vi "svl_Maximum Sound Level (1 Ch).vi"(6 "restart averaging (F)":bool, 8 "error in (no error)":errorcluster, 11 "energy level [dB]":waveform(dbl)={"t0"=timestamp(0 s since 1904-01-01), "dt"=0.0, "Y"=[]}) -> (0 "error out":errorcluster, 3 "maximum sound level [dB EU]":dbl format="%.2f")   [LabVIEW 2017]
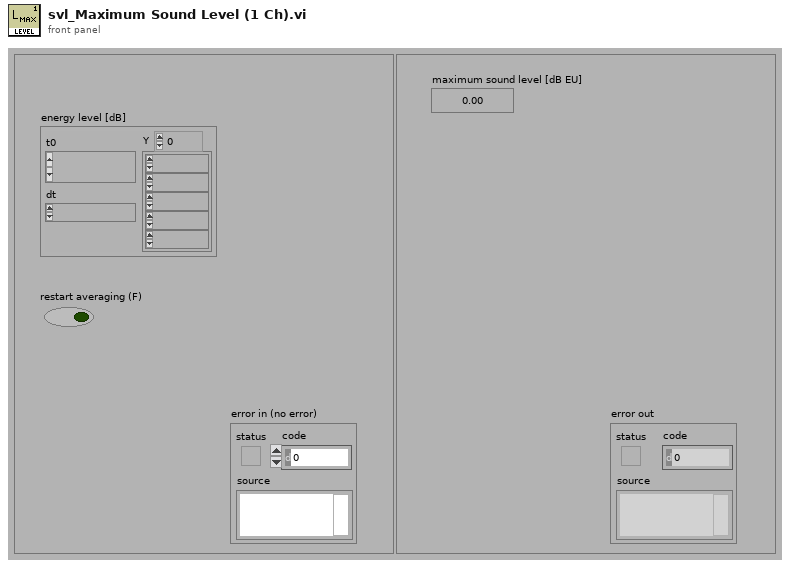
[diagram p1: front panel]
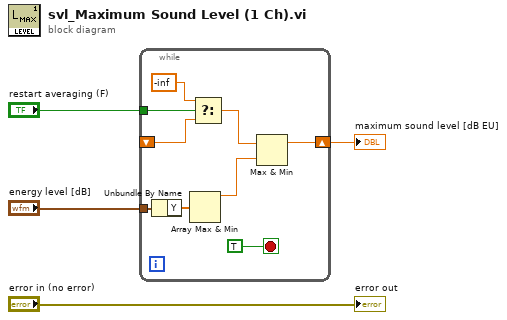
[diagram p0: block diagram]
diagram:
  n1 = while {
    shift-right: [w6] -> w2
    shift-left: _ -> [w11]
    tunnel: "restart averaging (F)" -> [w12]
    tunnel: "energy level [dB]" -> [w9]
    stop <- TRUE stop-if-true
    n2 = Unbundle By Name(w9) -> ("Y"=w5:dbl[])
    n3 = Array Max & Min(array=w5) -> (max value=w7:dbl)  [unwired: 3 out]
    n4 = Select(t=-inf ("maximum sound level [dB EU]"), s=w12, f=w11) -> (s? t:f=w8:dbl)
    n5 = Max & Min(x=w8, y=w7) -> (max(x,y)=w6:dbl)  [unwired: 1 out]
  }
  "maximum sound level [dB EU]" <- w2
  "error out" <- "error in (no error)"
